vi "view_shape.vi"() -> ()   [LabVIEW 2025]
panel:
  out "Waveform":dbl[](graph)
  in  "Data":string="array('I', [32768, 34957, 37136, 39295, 41425, 43517, 45560, 47547, 49467, 51313, 53076, 54748, 56322, 57791, 59149, 60388, 61504, 62492, 63346, 64065, 64643, 65080, 65371, 65518, 65518, 65371, 65080, 64643, 64065, 63346, 62492, 61504, 60388, 59149, 57791, 56322, 54748, 53076, 51313, 49467, 47547, 45560, 43517, 41425, 39295, 37136, 34957, 32768, 30579, 28400, 26241, 24111, 22019, 19976, 17989, 16069, 14223, 12460, 10788, 9214, 7745, 6387, 5148, 4032, 3044, 2190, 1471, 893, 456, 165, 18, 18, 165, 456, 893, 1471, 2190, 3044, 4032, 5148, 6387, 7745, 9214, 10788, 12460, 14223, 16069, 17989, 19976, 22019, 24111, 26241, 28401, 30579])"
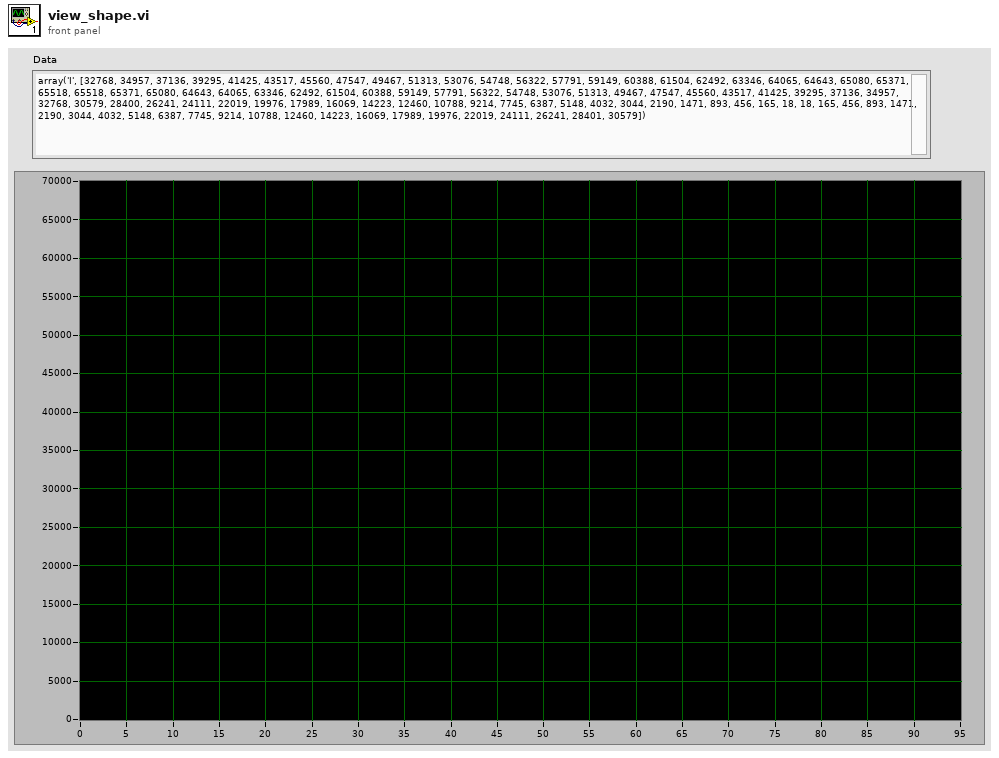
[diagram p1: front panel]
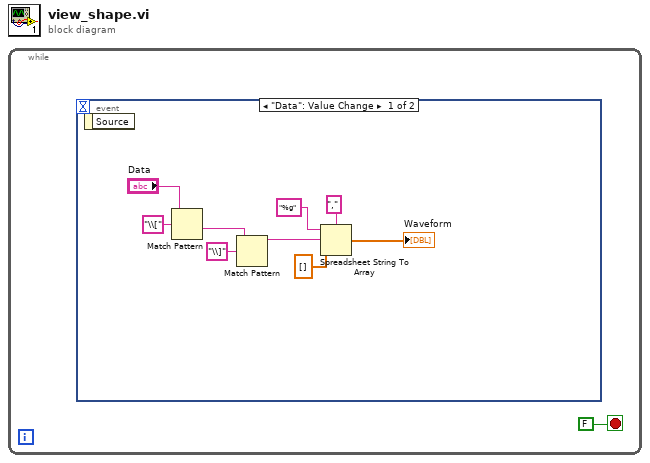
[diagram p0: block diagram]
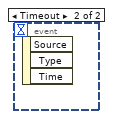
[diagram p2: hidden frame]
diagram:
  n1 = while {
    stop <- FALSE stop-if-true
    n2 = event shown="[0] \"Data\": Value Change" {
      selector: _ -> [_ _]
      dyn-events: _ -> [_ _]
      timeout: _ -> [_ _]
      event "Data": Value Change {
        n3 = event-data() -> ()  [unwired: 1 in, 1 out]
        n4 = Match Pattern(string="Data", regular expression="\\[") -> (after substring=w8:string)  [unwired: 1 in, 3 out]
        n5 = Match Pattern(string=w8, regular expression="\\]") -> (before substring=w6:string)  [unwired: 1 in, 3 out]
        n6 = Spreadsheet String To Array(delimiter (Tab)=",", format string="%g", spreadsheet string=w6, array type (2D Dbl)=dbl[] []) -> (array=→"Waveform":dbl[])
      }
      event Timeout {
        n7 = event-data() -> ()  [unwired: 1 in, 3 out]
      }
    }
  }
